vi "ELVIS III v1.0 AO Continuous Write.vi"(7 "Timeout":i32=-1 min=-1, 8 "error in (no error)":errorcluster, 9 "dbl Scaled Value List":dbl[][](array[numeric]), 10 "Channel Info":T1, 11 "myRIO Ref In":T2) -> (0 "error out":errorcluster, 2 "Channel InfoOut":T1, 3 "myRIO Ref Out":T2 caption="myRIO Ref In")   [LabVIEW 2021]
uses:
  <vilib>/myRIO/Common/Instrument Driver Framework/Utilities/typedefs/myRIO v1.0 Reference.ctl
  <vilib>/myRIO/Common/Instrument Driver Framework/Utilities/typedefs/Generic FPGA Reference.ctl
  <vilib>/myRIO/Common/Instrument Driver Framework/ELVIS III v1.0/AO Continuous/typedefs/AO Continuous Channel Info.ctl
  <vilib>/myRIO/Common/Instrument Driver Framework/ELVIS III v1.0/AO Block/typedefs/ELVIS III AO Block Channels FPGA Reference.ctl
  <vilib>/myRIO/Common/Instrument Driver Framework/myRIO v1.0/Resource Manager/vis/myRIO v1.0 Block Write Configuration.vi
  <vilib>/rvi/errors/niLvFpgaAdjustHostInterfaceError.vi
  <vilib>/rvi/interface/nirviReadWriteControl/nirviReadWriteControl.xnode
  <vilib>/rvi/interface/nirviMethod/nirviMethod.xnode
  <vilib>/FPGAPlugInAG/Dynamic/niLvFpga_WriteFifo_Dynamic.vi
  <vilib>/rvi/errors/niLvFpgaMergeErrorWithErrorCode.vi
  NiFpgaLv.dll
  <vilib>/rvi/interface/Simulation/niFpgaSimulationCallBeginRW.vi
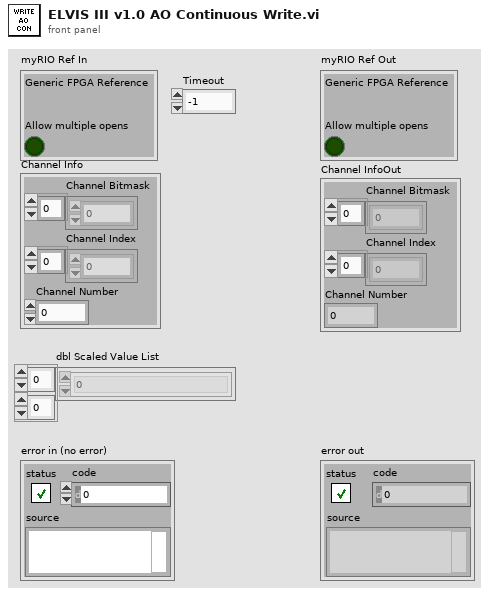
[diagram p1: front panel]
types:
  T1 = typedef "AO Continuous Channel Info.ctl" = cluster{"Channel Bitmask":u8[], "Channel Index":i32[], "Channel Number":u8}
  T2 = typedef "myRIO v1.0 Reference.ctl" = cluster{"Generic FPGA Reference":T3, "Allow multiple opens":bool}
  T3 = typedef "Generic FPGA Reference.ctl" = refnum<k20>
  T4 = typedef "ELVIS III AO Block Channels FPGA Reference.ctl" = refnum<k20>
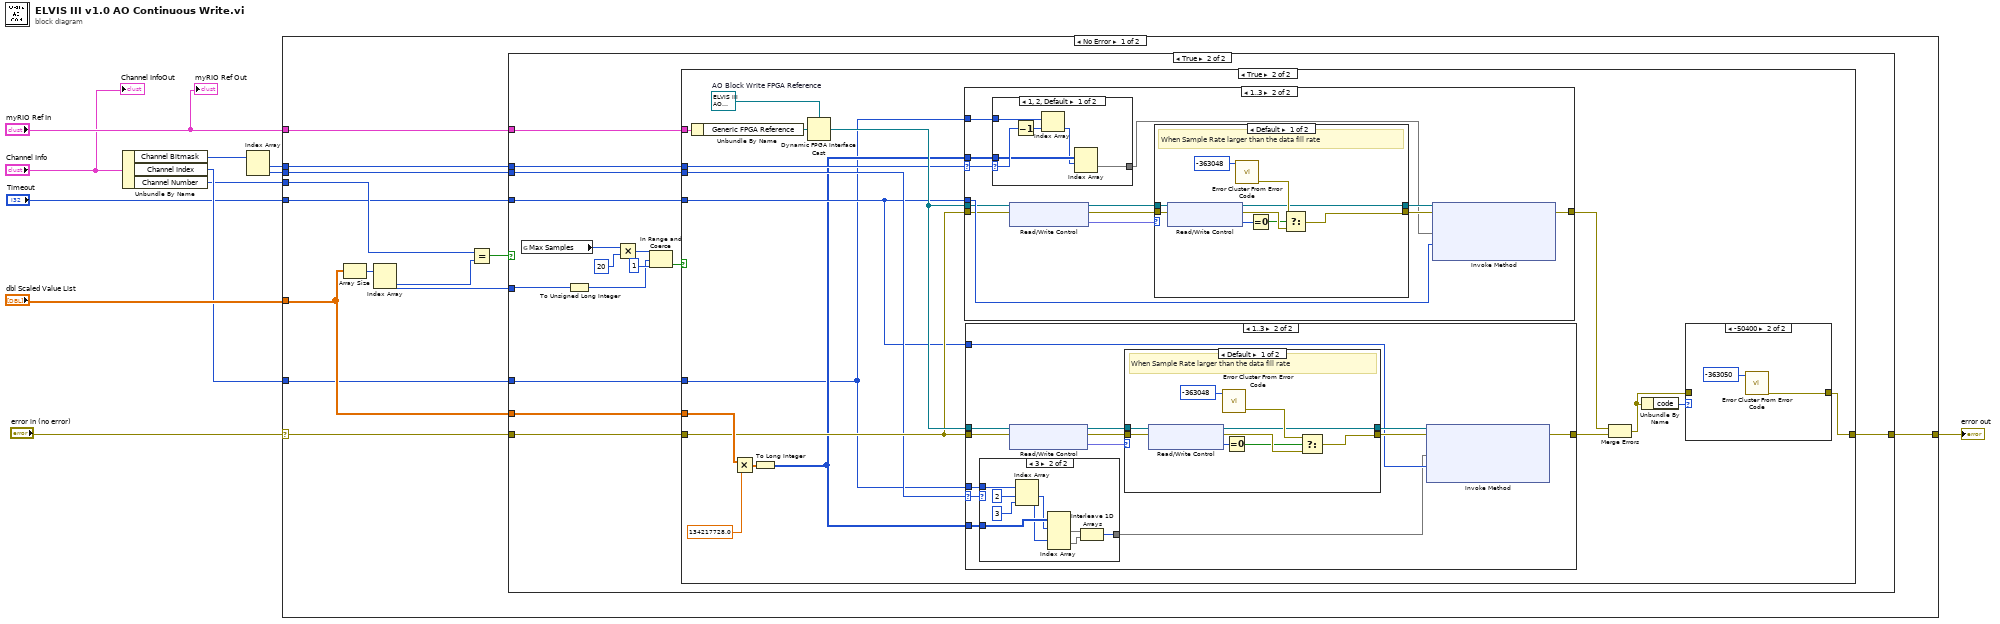
[diagram p0: block diagram]
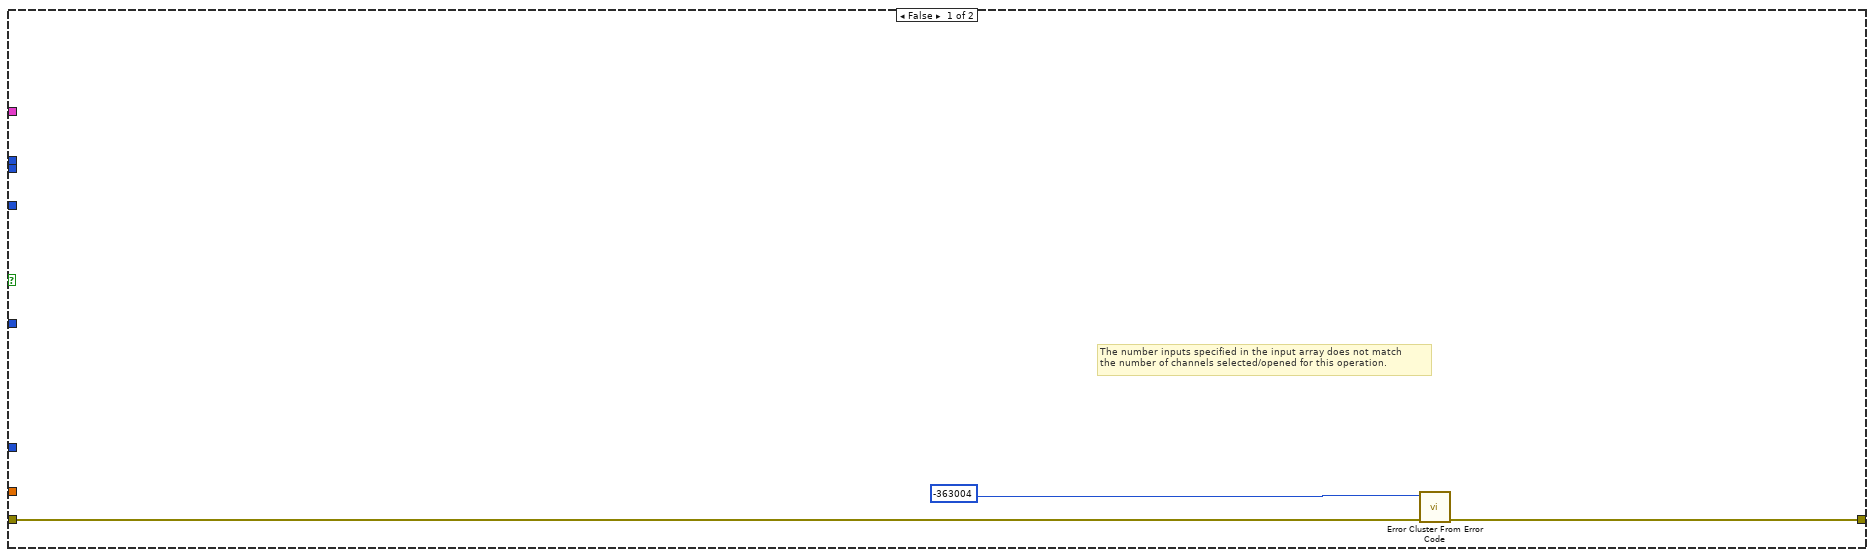
[diagram p2: hidden frame]
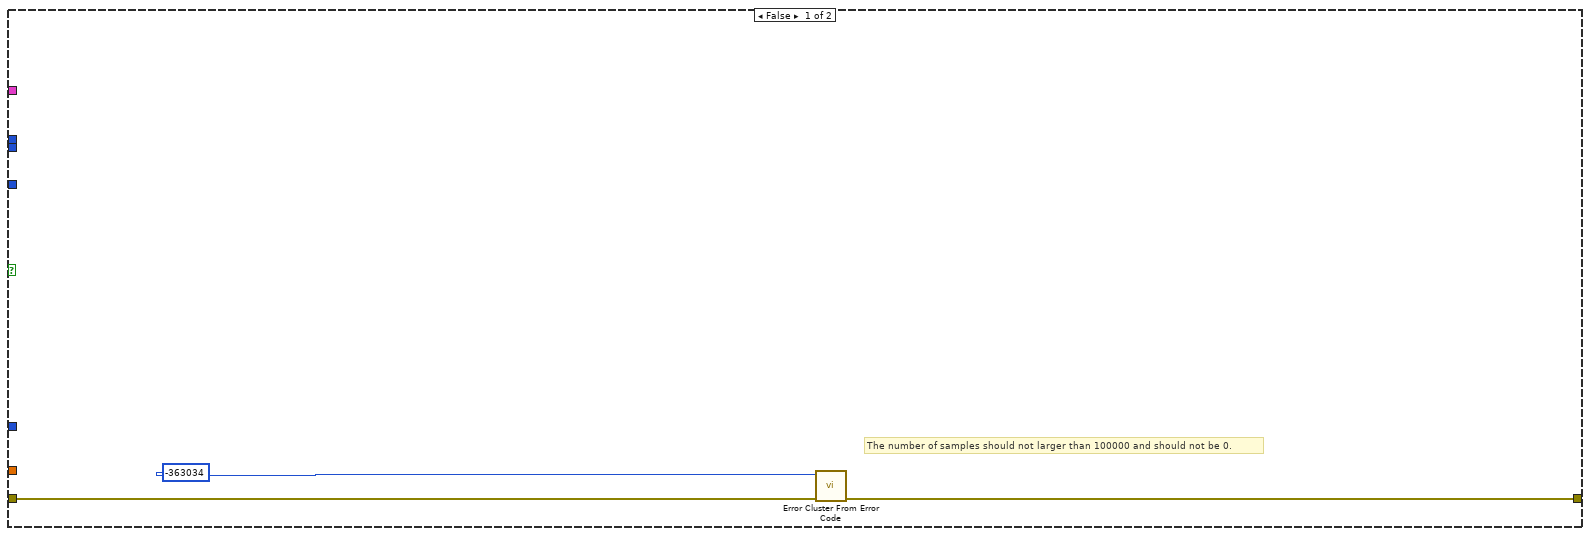
[diagram p3: hidden frame]
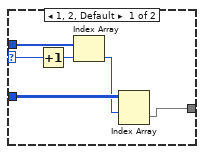
[diagram p6: hidden frame]
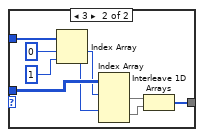
[diagram p9: hidden frame]
diagram:
  n1 = Unbundle By Name("Channel Info") -> ("Channel Bitmask"=w6:u8[], "Channel Index"=w3:i32[], "Channel Number"=w2:u8)
  n2 = Index Array(array=w6) -> (element #1=w5:u8, element #2=w4:u8)  [unwired: 2 in]
  n3 = case shown="No Error" "error in (no error)" {
    selector: "error in (no error)" -> [w21 w147]
    tunnel: w3 -> [w14 _]
    tunnel: "dbl Scaled Value List" -> [w19 _]
    tunnel: "myRIO Ref In" -> [w18 _]
    tunnel: w5 -> [w17 _]
    tunnel: w4 -> [w16 _]
    tunnel: [w15 w147] -> w9
    tunnel: w2 -> [w13 _]
    tunnel: "Timeout" -> [w12 _]
    frame No Error {
      n4 = Array Size(array=w19) -> (size(s)=w24:i32[])
      n5 = Index Array(array=w24) -> (element #1=w23:i32, element #2=w20:i32)  [unwired: 2 in]
      n6 = Equal?(x=w13, y=w23) -> (x = y?=w22:bool)
      n7 = case shown="True" w22 {
        tunnel: w21 -> [w27 w39]
        tunnel: w20 -> [_ w33]
        tunnel: w19 -> [_ w38]
        tunnel: w18 -> [_ w37]
        tunnel: w17 -> [_ w36]
        tunnel: w16 -> [_ w35]
        tunnel: [w26 w34] -> w15
        tunnel: w14 -> [_ w29]
        tunnel: w12 -> [_ w28]
        frame False {
          # "The number inputs specified in the input array does not match\nthe number of channels selected/opened for this operation."
          n8 = call <vilib>:"Error Cluster From Error Code.vi"("error in (no error)"=w27, "error code (0)"=-363004) -> ("error out"=w26:errorcluster)  [unwired: 7 in]
        }
        frame True {
          n9 = global read "myRIO v1.0 Block Write Configuration.vi" "Max Samples"() -> (w32:u32)
          n10 = To Unsigned Long Integer(number=w33) -> (unsigned 32bit integer=w41:u32)
          n11 = Multiply(x=w32, y=u32 20) -> (x*y=w30:u32)
          n12 = In Range and Coerce(upper limit=w30, x=w41, lower limit=u32 1) -> (In Range?=w40:bool)  [unwired: 1 out]
          n13 = case shown="True" w40 {
            tunnel: w39 -> [w44 w55]
            tunnel: [w43 w46] -> w34
            tunnel: w38 -> [_ w58]
            tunnel: w37 -> [_ w62]
            tunnel: w36 -> [_ w54]
            tunnel: w35 -> [_ w53]
            tunnel: w29 -> [_ w49]
            tunnel: w28 -> [_ w51]
            frame False {
              # "The number of samples should not larger than 100000 and should not be 0."
              n14 = call <vilib>:"Error Cluster From Error Code.vi"("error in (no error)"=w44, "error code (0)"=-363034) -> ("error out"=w43:errorcluster)  [unwired: 7 in]
            }
            frame True {
              w63 = T4 refnum  # AO Block Write FPGA Reference
              n15 = Unbundle By Name(w62) -> ("Generic FPGA Reference"=w61:T3)
              n16 = Multiply(x=w58, y=134217728.0) -> (x*y=w57:dbl[][])
              n17 = To Long Integer(number=w57) -> (32bit integer=w50:i32[][])
              n18 = Dynamic FPGA Interface Cast(Session In=w63, Type=w61) -> (Session Out=w56:T4)
              n19 = case shown="1..3" w54 {
                selector: w54 -> [_ w108]
                tunnel: w56 -> [_ w116]
                tunnel: w55 -> [w107 w115]
                tunnel: [w107 w118] -> w60
                tunnel: w51 -> [_ w117]
                tunnel: w50 -> [_ w110]
                tunnel: w49 -> [_ w109]
                frame Default {
                }
                frame 1..3 {
                  n20 = case shown="1, 2, Default" w108 {
                    selector: w108 -> [w126 _]
                    tunnel: [w124 w135] -> w111
                    tunnel: w110 -> [w125 w134]
                    tunnel: w109 -> [w122 w131]
                    frame 1, 2, Default {
                      n21 = Decrement(x=w126) -> (x-1=w123:u8)
                      n22 = Index Array(array=w122, index=w123) -> (element=w121:i32)
                      n23 = Index Array(array=w125, index (row)=w121) -> (element=w124:i32[])  [unwired: 1 in]
                    }
                    frame 3 {
                      n24 = Index Array(array=w131, index #1=0 ("index"), index #2=1 ("index")) -> (element #1=w128:i32, element #2=w127:i32)
                      n25 = Index Array(array=w134, index (row) #1=w128, index (row) #2=w127) -> (element #1=w133:i32[], element #2=w132:i32[])  [unwired: 2 in]
                      n26 = Interleave 1D Arrays(w133, w132) -> (w135:i32[])
                    }
                  }
                  n27 = xnode "Read/Write Control"("FPGA VI Reference In"=w116, "error in"=w115) -> ("FPGA VI Reference Out"=w114:T4, "error out"=w113:errorcluster, "AO.A.DMA_ENA"=w112:fxp<+,2,2>)
                  n28 = case shown="Default" w112 {
                    tunnel: w114 -> [w142 w145]
                    tunnel: w113 -> [w141 w146]
                    tunnel: [w138 w146] -> w119
                    tunnel: [w140 w145] -> w120
                    frame Default {
                      # "When Sample Rate larger than the data fill rate"
                      n29 = xnode "Read/Write Control"("FPGA VI Reference In"=w142, "error in"=w141) -> ("FPGA VI Reference Out"=w140:T4, "error out"=w139:errorcluster, "AO.A.ELE_NUM"=w137:u32)
                      n30 = call <vilib>:"Error Cluster From Error Code.vi"("error code (0)"=-363048) -> ("error out"=w143:errorcluster)  [unwired: 8 in]
                      n31 = Equal To 0?(x=w137) -> (x = 0?=w136:bool)
                      n32 = Select(t=w143, s=w136, f=w139) -> (s? t:f=w138:errorcluster)
                    }
                    frame 0 {
                      # "When Not Start the Generation"
                    }
                  }
                  n33 = xnode "Invoke Method"("FPGA VI Reference In"=w120, "error in"=w119, "Data"=w111, "Timeout (ms)"=w117) -> ("error out"=w118:errorcluster)  [unwired: 2 out]
                }
              }
              n34 = case shown="1..3" w53 {
                selector: w53 -> [_ w76]
                tunnel: w56 -> [_ w74]
                tunnel: w55 -> [w67 w72]
                tunnel: [w67 w78] -> w59
                tunnel: w51 -> [_ w77]
                tunnel: w50 -> [_ w69]
                tunnel: w49 -> [_ w68]
                frame Default {
                }
                frame 1..3 {
                  n35 = case shown="3" w76 {
                    selector: w76 -> [w86 _]
                    tunnel: [w84 w95] -> w75
                    tunnel: w69 -> [w85 w94]
                    tunnel: w68 -> [w82 w91]
                    frame 1, 2, Default {
                      n36 = Increment(x=w86) -> (x+1=w83:u8)
                      n37 = Index Array(array=w82, index=w83) -> (element=w81:i32)
                      n38 = Index Array(array=w85, index (row)=w81) -> (element=w84:i32[])  [unwired: 1 in]
                    }
                    frame 3 {
                      n39 = Index Array(array=w91, index #1=2 ("index"), index #2=3 ("index")) -> (element #1=w88:i32, element #2=w87:i32)
                      n40 = Index Array(array=w94, index (row) #1=w88, index (row) #2=w87) -> (element #1=w93:i32[], element #2=w92:i32[])  [unwired: 2 in]
                      n41 = Interleave 1D Arrays(w93, w92) -> (w95:i32[])
                    }
                  }
                  n42 = xnode "Read/Write Control"("FPGA VI Reference In"=w74, "error in"=w72) -> ("FPGA VI Reference Out"=w73:T4, "error out"=w71:errorcluster, "AO.B.DMA_ENA"=w70:fxp<+,2,2>)
                  n43 = case shown="Default" w70 {
                    tunnel: w73 -> [w99 w106]
                    tunnel: w71 -> [w98 w105]
                    tunnel: [w101 w105] -> w79
                    tunnel: [w100 w106] -> w80
                    frame Default {
                      # "When Sample Rate larger than the data fill rate"
                      n44 = xnode "Read/Write Control"("FPGA VI Reference In"=w99, "error in"=w98) -> ("FPGA VI Reference Out"=w100:T4, "error out"=w102:errorcluster, "AO.B.ELE_NUM"=w97:u32)
                      n45 = call <vilib>:"Error Cluster From Error Code.vi"("error code (0)"=-363048) -> ("error out"=w103:errorcluster)  [unwired: 8 in]
                      n46 = Equal To 0?(x=w97) -> (x = 0?=w96:bool)
                      n47 = Select(t=w103, s=w96, f=w102) -> (s? t:f=w101:errorcluster)
                    }
                    frame 0 {
                      # "When Not Start the Generation"
                    }
                  }
                  n48 = xnode "Invoke Method"("FPGA VI Reference In"=w80, "error in"=w79, "Data"=w75, "Timeout (ms)"=w77) -> ("error out"=w78:errorcluster)  [unwired: 2 out]
                }
              }
              n49 = Merge Errors(w60, w59) -> (w47:errorcluster)
              n50 = Unbundle By Name(w47) -> ("code"=w48:i32)
              n51 = case shown="-50400" w48 {
                tunnel: [w64 w65] -> w46
                tunnel: w47 -> [w64 _]
                frame Default {
                }
                frame -50400 {
                  n52 = call <vilib>:"Error Cluster From Error Code.vi"("error code (0)"=-363050) -> ("error out"=w65:errorcluster)  [unwired: 8 in]
                }
              }
            }
          }
        }
      }
    }
    frame Error {
    }
  }
  "error out" <- w9
  "myRIO Ref Out" <- "myRIO Ref In"
  "Channel InfoOut" <- "Channel Info"
